vi "Arduino Debug Settings Rd Wr.vi"(8 "error in (no error)":errorcluster, 10 "Write? (F:Read)":bool, 11 "Defaults":T1={"VISA resource name"="COM9", "Speed"=0, "Ramp Slope"=0, "Motor ID (0:n-1)"=0, "baud rate"=9600}) -> (0 "error out":errorcluster, 3 "Defaults":T1={"VISA resource name"="COM9", "Speed"=0, "Ramp Slope"=0, "Motor ID (0:n-1)"=0, "baud rate"=9600})   [LabVIEW 2024]
uses:
  Filter Wheel/Filter Wheel Arduino Control/Debug Program Settings.ctl
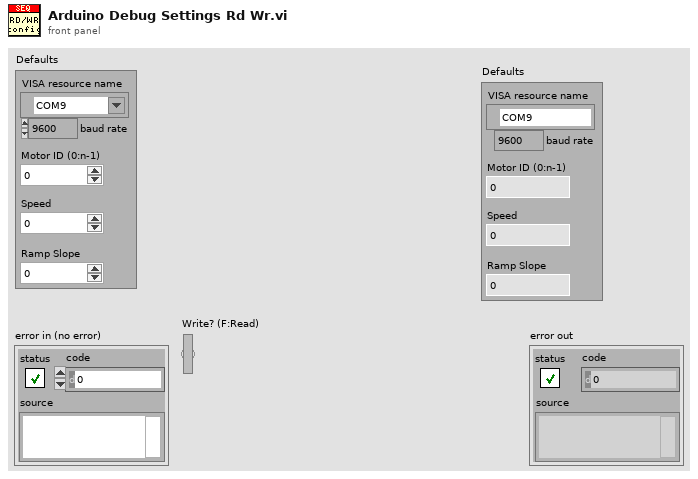
[diagram p1: front panel]
types:
  T1 = typedef "Debug Program Settings.ctl" = cluster{"VISA resource name":refnum<visa-resource-name>, "Speed":i32, "Ramp Slope":i32, "Motor ID (0:n-1)":i32, "baud rate":u32}
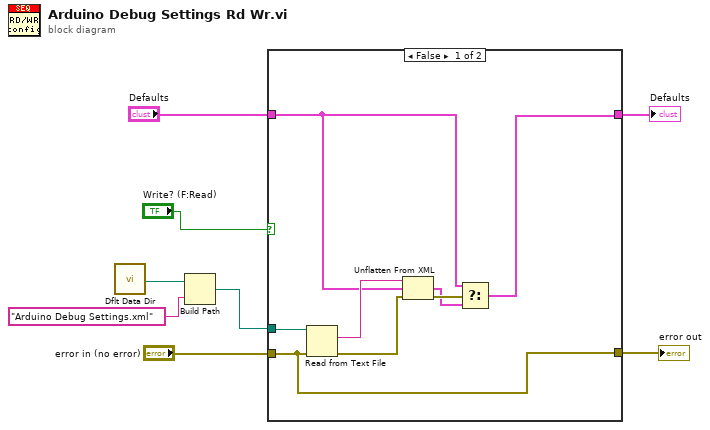
[diagram p0: block diagram]
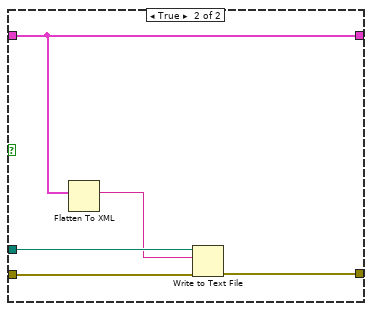
[diagram p2: hidden frame]
diagram:
  n1 = call <vilib>:"Dflt Data Dir.vi"() -> ("App:Default Data Directory"=w5:path)
  n2 = Build Path(base path=w5, name or relative path="Arduino Debug Settings.xml") -> (appended path=w4:path)
  n3 = case shown="False" "Write? (F:Read)" {
    tunnel: "error in (no error)" -> [w9 w21]
    tunnel: "Defaults" -> [w12 w17]
    tunnel: w4 -> [w16 w20]
    tunnel: [w9 w18] -> w3
    tunnel: [w10 w17] -> w2
    frame False {
      n4 = Read from Text File(file (use dialog)=w16, error in=w9) -> (text=w15:string, error out=w14:errorcluster)  [unwired: 2 in, 2 out]
      n5 = Unflatten From XML(xml string=w15, type=w12, error in (no error)=w14) -> (value=w11:T1, error out=w13:errorcluster)
      n6 = Select(t=w12, s=w13, f=w11) -> (s? t:f=w10:T1)
    }
    frame True {
      n7 = Flatten To XML(6:w17) -> (2:w19:string)
      n8 = Write to Text File(file (use dialog)=w20, text=w19, error in=w21) -> (error out=w18:errorcluster)  [unwired: 1 in, 2 out]
    }
  }
  "error out" <- w3
  "Defaults" <- w2
